vi "getAll.vi"(8 "error in (no error)":errorcluster, 11 "VoltageUpdate":refnum<class "VoltageUpdate.lvclass">) -> (0 "error out":errorcluster, 2 "getAll":variant, 3 "VoltageUpdate out":refnum<class "VoltageUpdate.lvclass">)   [LabVIEW 2016, in "VoltageUpdate.lvclass"]
uses:
  VoltageUpdate.lvclass
  VoltageUpdate.lvclass/VoltageUpdate.ctl
  <userlib>/LevyLab/Levylab Instruments/Instrument Types/VSource/Instrument.VSource.lvclass
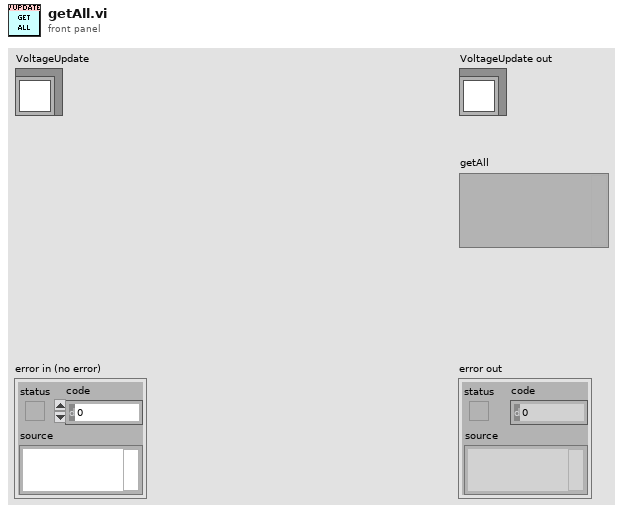
[diagram p1: front panel]
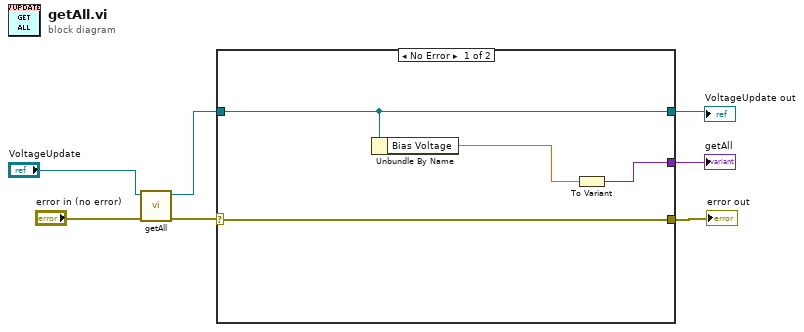
[diagram p0: block diagram]
diagram:
  n1 = call-parent "getAll.vi"("error in (no error)"="error in (no error)", "Instrument in"="VoltageUpdate") -> ("error out"=w5:errorcluster, "Instrument out"=w3:refnum<class "VoltageUpdate.lvclass">)  [unwired: 7 in, 1 out]
  n2 = case shown="No Error" w5 {
    selector: w5 -> [w11 w13]
    tunnel: [w11 w13] -> w4
    tunnel: w3 -> [w9 w12]
    tunnel: [w9 w12] -> w2
    tunnel: [w8 _] -> w1
    frame No Error {
      n3 = Unbundle By Name(w9) -> ("Bias Voltage"=w10:dbl)
      n4 = To Variant(anything=w10) -> (Variant=w8:variant)
    }
    frame Error {
    }
  }
  "error out" <- w4
  "VoltageUpdate out" <- w2
  "getAll" <- w1
